vi "Comm_Shutdown(SubVI).vi"(8 "error in (no error)":errorcluster) -> (0 "error out":errorcluster)   [LabVIEW 2018, in "MainFrameLib.lvlib"]
uses:
  MainFrameLib.lvlib
  TypeDefs/FGV_Enum.ctl
  TypeDefs/Command_Enum.ctl
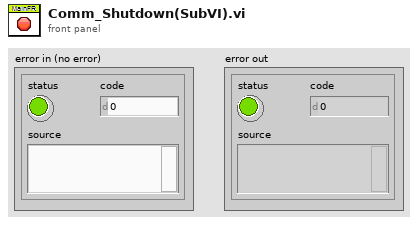
[diagram p1: front panel]
types:
  T1 = typedef "MainFrameLib.lvlib/FGV_Enum.ctl" = enum16{"Close", "GetRefs", "Initialize"}
  T2 = typedef "MainFrameLib.lvlib/Command_Enum.ctl" = enum16{"CheckSRLinks", "UpdateKCSColorCode", "StartLinkageCheck", "GetSRNotes", "DisplayAEStats", "InWork&Neglected", "RemapAENames", "ClearFolder", "UpdateReportsList", "ExcelReports", "TeamStats", "LoadReport", "WaitOnReport", "RequestReport", "Error", "Idle", "InitializeData", "ScreenPop", "Initialize", "UpdateCiscoAgentsView", "CancelRequests", "ClipboardCopy", "SaveNeglectedToFile", "Shutdown"}
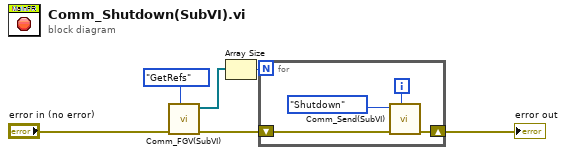
[diagram p0: block diagram]
diagram:
  n1 = call "Comm_FGV(SubVI).vi"("Enum"=FGV_Enum."GetRefs", "error in (no error)"="error in (no error)") -> ("error out"=w5:errorcluster, "Array"=w3:refnum<queue>[])  [unwired: 8 in]
  n2 = Array Size(array=w3) -> (size(s)=w4:i32)
  n3 = for {
    N: w4 -> [_]
    shift-right: [w8] -> w6
    shift-left: w5 -> [w9]
    i -> [w7]
    n4 = call "Comm_Send(SubVI).vi"("QueuSelector"=w7, "Error In"=w9, "Command"=Command_Enum."Shutdown") -> ("error out"=w8:errorcluster)  [unwired: 8 in]
  }
  "error out" <- w6
